vi "Open.vi"(7 "Allow multiple opens?":bool, 8 "error in (no error)":errorcluster, 10 "Channel Names":tag[](array[tag])) -> (0 "error out":errorcluster, 3 "DI (N Samples) Ref Out":T1)   [LabVIEW 2021, in "DI Block.lvlib"]
doc: "Opens a reference to the digital input block read channel (ConnectorA/DIO0). You must open a reference before you read values."
uses:
  <vilib>/myRIO/Instrument Drivers/Onboard IO/DI Block/DI Block.lvlib
  <vilib>/myRIO/Instrument Drivers/Onboard IO/DI Block/typedefs/DI Block Reference.ctl
  <vilib>/myRIO/Common/Instrument Driver Framework/Utilities/typedefs/myRIO Generic Hardware Reference.ctl
  <vilib>/myRIO/Common/Instrument Driver Framework/Utilities/typedefs/Hardware Version Enum.ctl
  <vilib>/myRIO/Common/Instrument Driver Framework/Utilities/typedefs/myRIO v1.0 Reference.ctl
  <vilib>/myRIO/Common/Instrument Driver Framework/Utilities/typedefs/Generic FPGA Reference.ctl
  <vilib>/myRIO/Common/Instrument Driver Framework/myRIO v1.0/DI Block/typedefs/DI Block Channels List.ctl
  <vilib>/myRIO/Common/Instrument Driver Framework/myRIO v1.0/DI Block/typedefs/DI Block Channels Enum.ctl
  <vilib>/userdefined/High Color/nirio_resource_hc.ctl
panel:
  # "DI (N Samples) Open"
  # "Opens a reference to the myRIO hardware and configures the DI (N Samples) Reference with channels to be read"
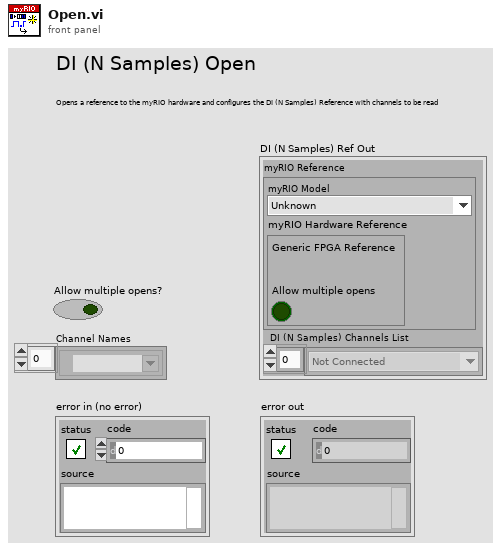
[diagram p1: front panel]
types:
  T1 = typedef "DI Block.lvlib/DI Block Reference.ctl" = cluster{"myRIO Reference":T2, "DI (N Samples) Channels List":T6}
  T2 = typedef "myRIO Generic Hardware Reference.ctl" = cluster{"myRIO Model":T3, "myRIO Hardware Reference":T4}
  T3 = typedef "Hardware Version Enum.ctl" = enum16{"Unknown", "myRIO-1900", "myRIO-1950", "roboRIO", "NI ELVIS RIO CM", "ELVIS III"}
  T4 = typedef "myRIO v1.0 Reference.ctl" = cluster{"Generic FPGA Reference":T5, "Allow multiple opens":bool}
  T5 = typedef "Generic FPGA Reference.ctl" = refnum<k20>
  T6 = typedef "DI Block Channels List.ctl" = T7[]
  T7 = typedef "DI Block Channels Enum.ctl" = enum16{"Not Connected", "A/DI0 (N Samples)", "A/DI1 (N Samples)", "A/DI2 (N Samples)", "A/DI3 (N Samples)", "A/DI4 (N Samples)", "A/DI5 (N Samples)", "A/DI6 (N Samples)", "A/DI7 (N Samples)", "A/DI8 (N Samples)", "A/DI9 (N Samples)", "A/DI10 (N Samples)", "A/DI11 (N Samples)", "A/DI12 (N Samples)", "A/DI13 (N Samples)", "A/DI14 (N Samples)", "A/DI15 (N Samples)", "A/DI16 (N Samples)", "A/DI17 (N Samples)", "A/DI18 (N Samples)", "A/DI19 (N Samples)", "B/DI0 (N Samples)", "B/DI1 (N Samples)", "B/DI2 (N Samples)", "B/DI3 (N Samples)", "B/DI4 (N Samples)", "B/DI5 (N Samples)", "B/DI6 (N Samples)", "B/DI7 (N Samples)", "B/DI8 (N Samples)", "B/DI9 (N Samples)", "B/DI10 (N Samples)", "B/DI11 (N Samples)", "B/DI12 (N Samples)", "B/DI13 (N Samples)", "B/DI14 (N Samples)", "B/DI15 (N Samples)", "B/DI16 (N Samples)", "B/DI17 (N Samples)", "B/DI18 (N Samples)", "B/DI19 (N Samples)"}
  T8 = typedef "nirio_resource_hc.ctl" = tag
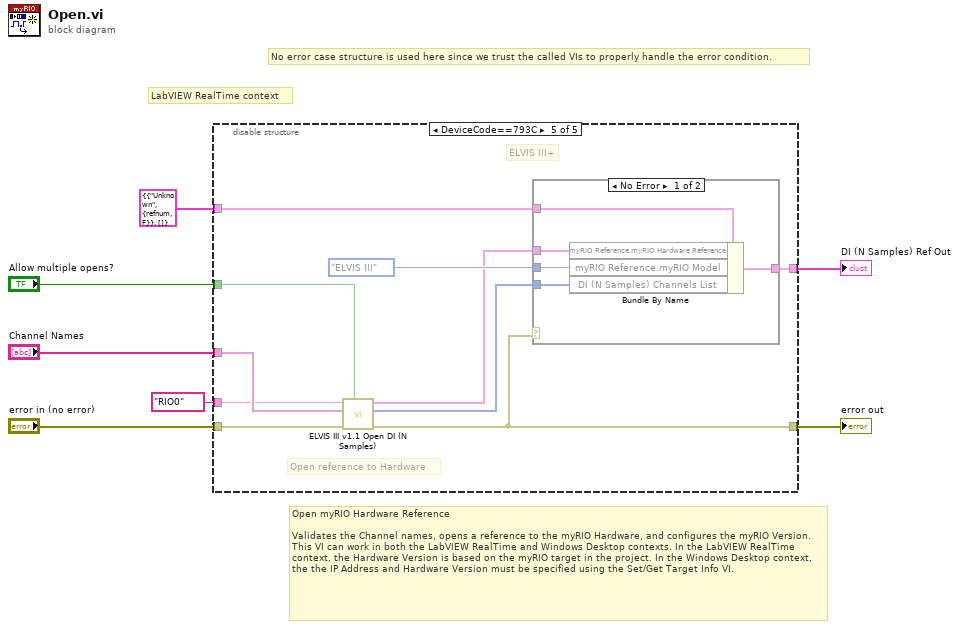
[diagram p0: block diagram]
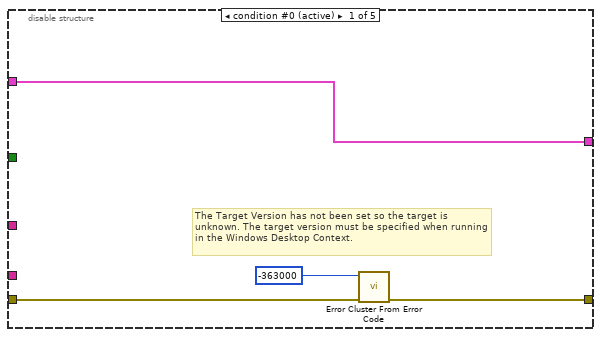
[diagram p2: hidden frame]
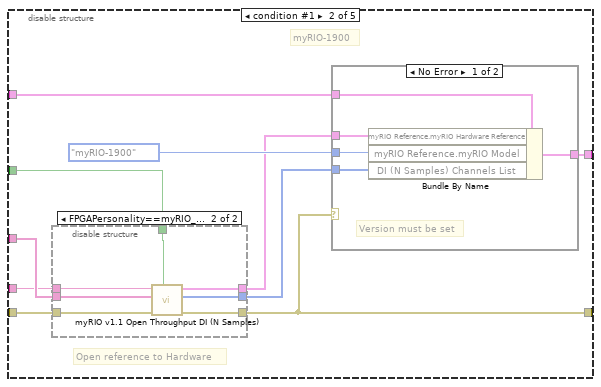
[diagram p3: hidden frame]
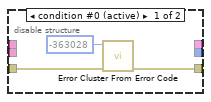
[diagram p4: hidden frame]
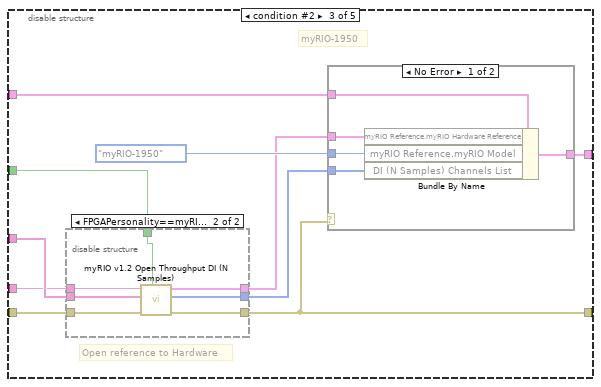
[diagram p6: hidden frame]
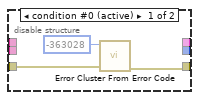
[diagram p7: hidden frame]
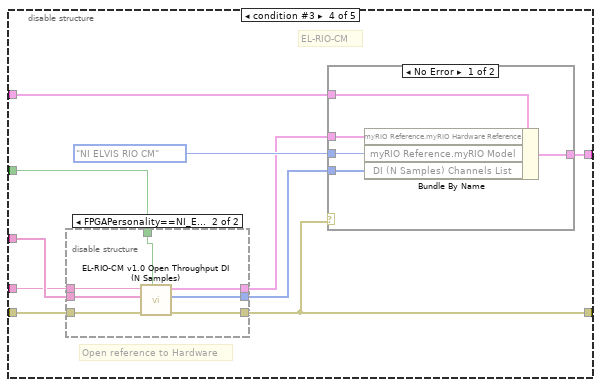
[diagram p9: hidden frame]
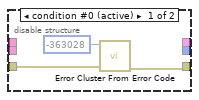
[diagram p10: hidden frame]
diagram:
  # "LabVIEW RealTime context"
  # "No error case structure is used here since we trust the called VIs to properly handle the error condition."
  # "Open myRIO Hardware Reference\n\nValidates the Channel names, opens a reference to the myRIO Hardware, and configures the myRIO Version. This VI can work in both the LabVIEW RealTime and Windows Desktop contexts. In the LabVIEW RealTime context, the Hardware Version is based on the myRIO target in the project. In the Windows Desktop context, the the IP Address and Hardware Version must be specified using the Set/Get Target Info VI."
  n1 = disable-structure shown="DeviceCode==793C" {
    disable-tunnel: [w11 w13 w39 w65 w91] -> w4
    disable-tunnel: "Channel Names" -> [_ w21 w47 w73 w94]
    disable-tunnel: "Allow multiple opens?" -> [_ w17 w46 w72 w95]
    disable-tunnel: [w8 w20 w45 w71 w90] -> w1
    disable-tunnel: "error in (no error)" -> [w10 w18 w43 w69 w92]
    disable-tunnel: T1 {"myRIO Reference"={"myRIO Model"=enum."Unknown", "myRIO Hardware Reference"={"Generic FPGA Reference"=refnum, "Allow multiple opens"=FALSE}}, "DI (N Samples) Channels List"=[]} ("DI Block Read Ref Out") -> [w8 w16 w41 w67 w96]
    disable-tunnel: T8 "RIO0" ("Resource name") -> [_ w14 w40 w66 w93]
    frame condition #0 (active) {
      # "The Target Version has not been set so the target is unknown. The target version must be specified when running in the Windows Desktop Context."
      n2 = call <vilib>:"Error Cluster From Error Code.vi"("error in (no error)"=w10, "error code (0)"=-363000) -> ("error out"=w11:errorcluster)  [unwired: 7 in]
    }
    frame condition #1 {
      # "myRIO-1900"
      # "Open reference to Hardware"
      n3 = disable-structure shown="FPGAPersonality==myRIO_FP_Throughput" {
        disable-tunnel: w21 -> [_ w29]
        disable-tunnel: w18 -> [w23 w28]
        disable-tunnel: w17 -> [_ w31]
        disable-tunnel: [_ w26] -> w15
        disable-tunnel: w14 -> [_ w30]
        disable-tunnel: [w22 w25] -> w13
        disable-tunnel: [_ w27] -> w12
        frame condition #0 (active) {
          n4 = call <vilib>:"Error Cluster From Error Code.vi"("error in (no error)"=w23, "error code (0)"=-363028) -> ("error out"=w22:errorcluster)  [unwired: 7 in]
        }
        frame condition #1 {
          n5 = call <vilib>:"myRIO v1.1 Open Throughput DI (N Samples).vi"("Allow multiple opens?"=w31, "error in (no error)"=w28, "Channel Names"=w29, "Resource name"=w30) -> ("error out"=w25:errorcluster, "DI (N Samples) Channel List"=w26:T6, "myRIO Ref Out"=w27:T4)  [unwired: 5 in]
        }
      }
      n6 = case shown="No Error" w13 {
        tunnel: [w36 w37] -> w20
        tunnel: Hardware_Version_Enum."myRIO-1900" ("Hardware Version Enum") -> [w35 _]
        tunnel: w16 -> [w34 w37]
        tunnel: w15 -> [w32 _]
        tunnel: w12 -> [w33 _]
        frame No Error {
          # "Version must be set"
          n7 = Bundle By Name(cluster=w34, "myRIO Reference.myRIO Hardware Reference"=w33, "myRIO Reference.myRIO Model"=w35, "DI (N Samples) Channels List"=w32) -> (w36:T1)
        }
        frame Error {
        }
      }
    }
    frame condition #2 {
      # "myRIO-1950"
      # "Open reference to Hardware"
      n8 = disable-structure shown="FPGAPersonality==myRIO_FP_Throughput" {
        disable-tunnel: w47 -> [_ w55]
        disable-tunnel: w46 -> [_ w57]
        disable-tunnel: w43 -> [w49 w54]
        disable-tunnel: [_ w53] -> w42
        disable-tunnel: w40 -> [_ w56]
        disable-tunnel: [w48 w51] -> w39
        disable-tunnel: [_ w52] -> w38
        frame condition #0 (active) {
          n9 = call <vilib>:"Error Cluster From Error Code.vi"("error in (no error)"=w49, "error code (0)"=-363028) -> ("error out"=w48:errorcluster)  [unwired: 7 in]
        }
        frame condition #1 {
          n10 = call <vilib>:"myRIO v1.2 Open Throughput DI (N Samples).vi"("Allow multiple opens?"=w57, "error in (no error)"=w54, "Channel Names"=w55, "Resource name"=w56) -> ("error out"=w51:errorcluster, "DI (N Samples) Channel List"=w52:T6, "myRIO Ref Out"=w53:T4)  [unwired: 5 in]
        }
      }
      n11 = case shown="No Error" w39 {
        tunnel: [w62 w63] -> w45
        tunnel: Hardware_Version_Enum."myRIO-1950" ("Hardware Version Enum") -> [w61 _]
        tunnel: w42 -> [w58 _]
        tunnel: w41 -> [w60 w63]
        tunnel: w38 -> [w59 _]
        frame No Error {
          n12 = Bundle By Name(cluster=w60, "myRIO Reference.myRIO Hardware Reference"=w58, "myRIO Reference.myRIO Model"=w61, "DI (N Samples) Channels List"=w59) -> (w62:T1)
        }
        frame Error {
        }
      }
    }
    frame condition #3 {
      # "EL-RIO-CM"
      # "Open reference to Hardware"
      n13 = disable-structure shown="FPGAPersonality==NI_ELVIS_RIO_CM_FP_Throughput" {
        disable-tunnel: w73 -> [_ w81]
        disable-tunnel: w72 -> [_ w83]
        disable-tunnel: w69 -> [w75 w80]
        disable-tunnel: [_ w79] -> w68
        disable-tunnel: w66 -> [_ w82]
        disable-tunnel: [w74 w77] -> w65
        disable-tunnel: [_ w78] -> w64
        frame condition #0 (active) {
          n14 = call <vilib>:"Error Cluster From Error Code.vi"("error in (no error)"=w75, "error code (0)"=-363028) -> ("error out"=w74:errorcluster)  [unwired: 7 in]
        }
        frame condition #1 {
          n15 = call <vilib>:"EL-RIO-CM v1.0 Open Throughput DI (N Samples).vi"("Allow multiple opens?"=w83, "error in (no error)"=w80, "Channel Names"=w81, "Resource name"=w82) -> ("error out"=w77:errorcluster, "DI (N Samples) Channel List"=w78:T6, "myRIO Ref Out"=w79:T4)  [unwired: 5 in]
        }
      }
      n16 = case shown="No Error" w65 {
        tunnel: [w88 w89] -> w71
        tunnel: Hardware_Version_Enum."NI ELVIS RIO CM" ("Hardware Version Enum") -> [w87 _]
        tunnel: w68 -> [w84 _]
        tunnel: w67 -> [w86 w89]
        tunnel: w64 -> [w85 _]
        frame No Error {
          n17 = Bundle By Name(cluster=w86, "myRIO Reference.myRIO Hardware Reference"=w84, "myRIO Reference.myRIO Model"=w87, "DI (N Samples) Channels List"=w85) -> (w88:T1)
        }
        frame Error {
        }
      }
    }
    frame condition #4 {
      # "ELVIS III+"
      # "Open reference to Hardware"
      n18 = call <vilib>:"ELVIS III v1.1 Open DI (N Samples).vi"("Allow multiple opens?"=w95, "error in (no error)"=w92, "Channel Names"=w94, "Resource name"=w93) -> ("error out"=w91:errorcluster, "DI (N Samples) Channel List"=w97:T6, "myRIO Ref Out"=w98:T4)  [unwired: 5 in]
      n19 = case shown="No Error" w91 {
        tunnel: [w104 w105] -> w90
        tunnel: Hardware_Version_Enum."ELVIS III" ("Hardware Version Enum") -> [w103 _]
        tunnel: w98 -> [w100 _]
        tunnel: w96 -> [w102 w105]
        tunnel: w97 -> [w101 _]
        frame No Error {
          n20 = Bundle By Name(cluster=w102, "myRIO Reference.myRIO Hardware Reference"=w100, "myRIO Reference.myRIO Model"=w103, "DI (N Samples) Channels List"=w101) -> (w104:T1)
        }
        frame Error {
        }
      }
    }
  }
  "DI (N Samples) Ref Out" <- w1
  "error out" <- w4
